vi "Rename Window Title to VI Name.vi"(8 "error in (no error)":errorcluster, 11 "vi path":path) -> (0 "error out":errorcluster)   [LabVIEW 2023]
uses:
  <userlib>/_OpenG.lib/file/file.llb/Strip Path Extension - String__ogtk.vi
  <userlib>/_OpenG.lib/file/file.llb/openg_file.lvlib
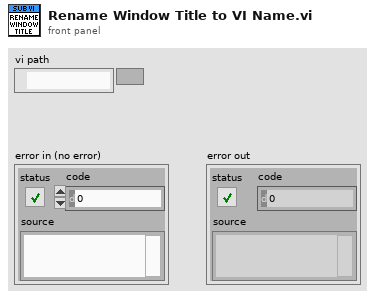
[diagram p1: front panel]
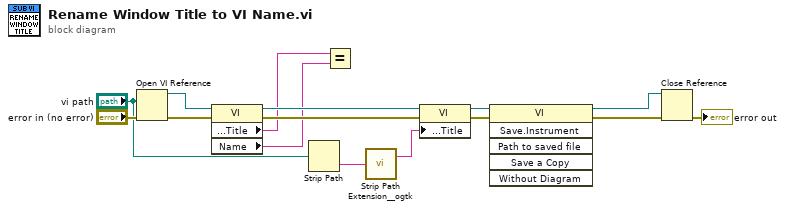
[diagram p0: block diagram]
diagram:
  n1 = Open VI Reference(vi path="vi path", error in (no error)="error in (no error)") -> (vi reference=w12:refnum<vi>, error out=w11:errorcluster)  [unwired: 4 in]
  n2 = property class="VI"(reference=w12, error in=w11) -> (reference out=w15:refnum<vi>, error out=w14:errorcluster, "Front Panel.Title"=w10:string, "Name"=w9:string)
  n3 = Strip Path(path="vi path") -> (name=w2:string)  [unwired: 1 out]
  n4 = Equal?(x=w10, y=w9) -> ()  [unwired: 1 out]
  n5 = call-poly <userlib>:"Strip Path Extension__ogtk.vi"("path"=w2) -> ("root"=w1:string)  [unwired: 1 out]
  n6 = property class="VI"(reference=w15, error in=w14, "Front Panel.Title"=w1) -> (reference out=w5:refnum<vi>, error out=w4:errorcluster)
  n7 = invoke class="VI" method="Save.Instrument"(reference=w5, error in=w4) -> (reference out=w7:refnum<vi>, error out=w8:errorcluster)  [unwired: 4 in, 4 out]
  n8 = Close Reference(reference=w7, error in (no error)=w8) -> (error out=→"error out":errorcluster)
